vi "Updated4x7Display.vi"(8 "Error In":errorcluster, 10 "Cluster":cluster{"Score":u32, "Time":u32, "Combo":u32}={"Score"=4, "Time"=4, "Combo"=4}, 11 "LINX Resource In":T1) -> (0 "Error Out":errorcluster, 3 "LINX Resource Out":T1)   [LabVIEW 2022 SP3]
doc: "Custom Command 7 is for the Score Display. Custom Command 8 is for the Time Display. Custom Command 9 is for Combo Display. Sends number to display to the applicable 7 segment display."
uses:
  <vilib>/MakerHub/LINX/Private/Type Defs/LINX Ref.ctl
  <vilib>/MakerHub/LINX/Private/Type Defs/Platform.ctl
  <vilib>/MakerHub/LINX/Private/Type Defs/Interface.ctl
  <vilib>/MakerHub/LINX/Private/Device/Type Defs/LINX Device Config.ctl
  <vilib>/MakerHub/LINX/Private/Device/Type Defs/TCP Config.ctl
  <vilib>/MakerHub/LINX/Private/Device/Type Defs/Channels.ctl
  <vilib>/MakerHub/LINX/LMH-LINX.lvlib
  <vilib>/MakerHub/LINX/Private/Device/Device.lvlib
panel:
  out "Response":u8[](array[numeric])
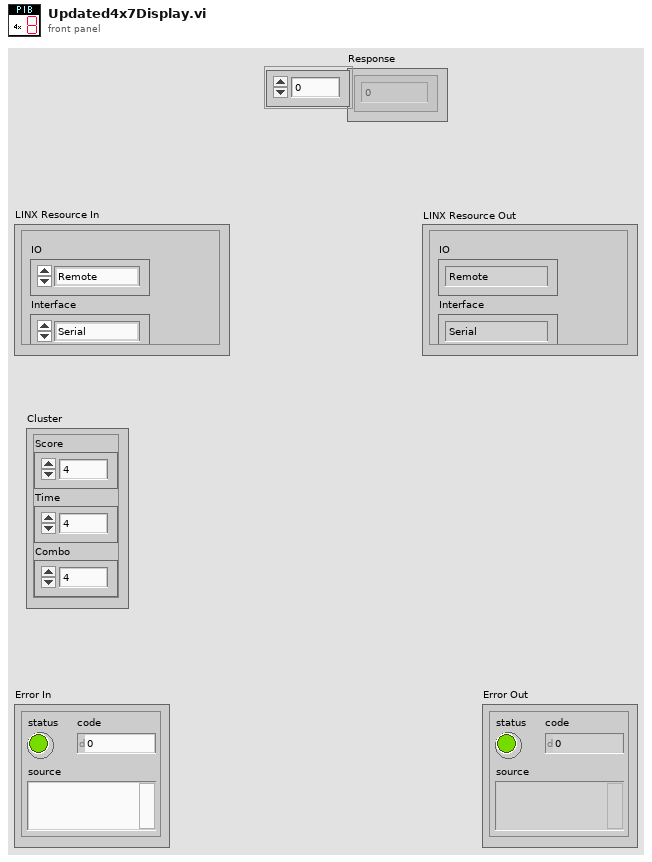
[diagram p1: front panel]
types:
  T1 = typedef "LMH-LINX.lvlib/LINX Ref.ctl" = cluster{"IO":T2, "Interface":T3, "LINX Device Config":T4}
  T2 = typedef "LMH-LINX.lvlib/Platform.ctl" = enum16{"Remote", "Local"}
  T3 = typedef "LMH-LINX.lvlib/Interface.ctl" = enum16{"Serial", "TCP"}
  T4 = typedef "LMH-LINX.lvlib/Device.lvlib/LINX Device Config.ctl" = cluster{"Interface":T3, "COM Port":refnum<visa-resource-name>, "TCP Configuration":T5, "Device Family":u8, "Device ID":u8, "Device Name":string, "TCP Ref":refnum<k5>, "Channels":T6}
  T5 = typedef "LMH-LINX.lvlib/Device.lvlib/TCP Config.ctl" = cluster{"IP Address":string, "Port":u16}
  T6 = typedef "LMH-LINX.lvlib/Channels.ctl" = cluster{"DI":u8[], "DO":u8[], "AI":u8[], "AO":u8[], "PWM":u8[], "QE":u8[], "UART":u8[], "I2C 2":u8[], "SPI":u8[], "CAN":u8[], "Servo":u8[], "AI Ref (V)":dbl, "AI Resolution (Bits)":u8, "AO Ref (V)":dbl, "AO Resolution (Bits)":u8}
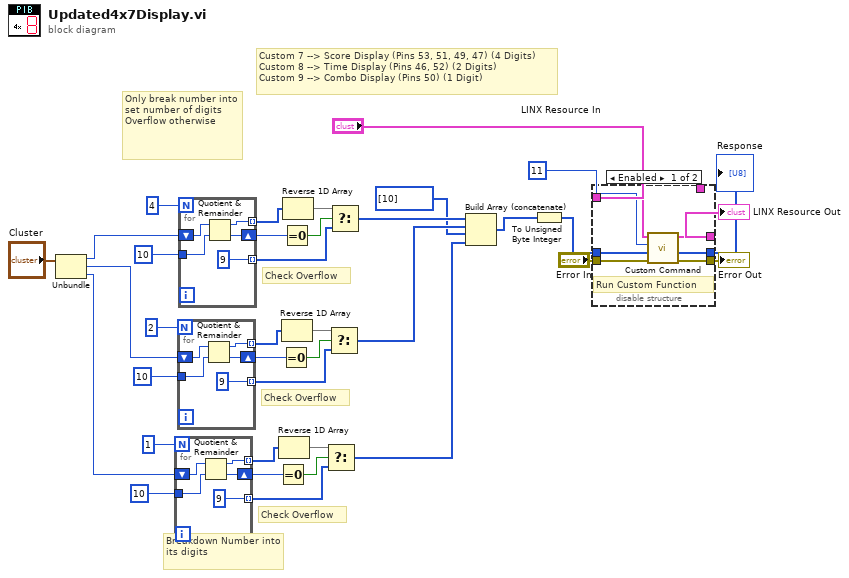
[diagram p0: block diagram]
diagram:
  # "Check Overflow"
  # "Check Overflow"
  # "Check Overflow"
  # "Breakdown Number into its digits"
  # "Custom 7 --> Score Display (Pins 53, 51, 49, 47) (4 Digits)\nCustom 8 --> Time Display (Pins 46, 52) (2 Digits)\nCustom 9 --> Combo Display (Pins 50) (1 Digit)"
  # "Only break number into set number of digits\nOverflow otherwise"
  n1 = Unbundle("Cluster") -> ("Score"=w31:u32, "Time"=w30:u32, "Combo"=w29:u32)
  n2 = for {
    N: 1 ("Display Length") -> [_]
    tunnel: u32 10 -> [w38]
    tunnel: [w40] -> w6 mode=indexing
    tunnel: [u32 9] -> w7 mode=indexing
    shift-right: [w41] -> w5
    shift-left: w29 -> [w42]
    n3 = Quotient & Remainder(x=w42, y=w38) -> (x-y*floor(x/y)=w40:u32, floor(x/y)=w41:u32)
  }
  n4 = for {
    N: 2 ("Display Length") -> [_]
    tunnel: u32 10 -> [w43]
    tunnel: [w45] -> w13 mode=indexing
    tunnel: [u32 9] -> w14 mode=indexing
    shift-right: [w46] -> w12
    shift-left: w30 -> [w47]
    n5 = Quotient & Remainder(x=w47, y=w43) -> (x-y*floor(x/y)=w45:u32, floor(x/y)=w46:u32)
  }
  n6 = for {
    N: 4 ("Display Length") -> [_]
    tunnel: u32 10 -> [w48]
    tunnel: [w50] -> w20 mode=indexing
    tunnel: [u32 9] -> w21 mode=indexing
    shift-right: [w51] -> w19
    shift-left: w31 -> [w52]
    n7 = Quotient & Remainder(x=w52, y=w48) -> (x-y*floor(x/y)=w50:u32, floor(x/y)=w51:u32)
  }
  n8 = Equal To 0?(x=w5) -> (x = 0?=w8:bool)
  n9 = Reverse 1D Array(array=w6) -> (reversed array=w9:u32[])
  n10 = Equal To 0?(x=w12) -> (x = 0?=w15:bool)
  n11 = Equal To 0?(x=w19) -> (x = 0?=w22:bool)
  n12 = Reverse 1D Array(array=w13) -> (reversed array=w16:u32[])
  n13 = Reverse 1D Array(array=w20) -> (reversed array=w23:u32[])
  n14 = Select(t=w9, s=w8, f=w7) -> (s? t:f=w2:u32[])
  n15 = Select(t=w16, s=w15, f=w14) -> (s? t:f=w24:u32[])
  n16 = Select(t=w23, s=w22, f=w21) -> (s? t:f=w25:u32[])
  n17 = Build Array (concatenate)(w25, w24, u32[] [10] ("array"), w2) -> (w28:u32[])
  n18 = To Unsigned Byte Integer(number=w28) -> (unsigned 8bit integer=w36:u8[])
  n19 = disable-structure shown="Enabled" {
    disable-tunnel: u16 11 ("Custom Command Number") -> [w59 _]
    disable-tunnel: w36 -> [w58 w61]
    disable-tunnel: "LINX Resource In" -> [w57 _]
    disable-tunnel: [w56 w62] -> w35
    disable-tunnel: "Error In" -> [w55 w60]
    disable-tunnel: [w54 w60] -> w33
    disable-tunnel: [w53 w61] -> w27
    disable-tunnel: "LINX Resource In" -> [_ w62]
    frame Enabled {
      # "Run Custom Function"
      n20 = call <vilib>:"Custom Command.vi"("Error In"=w55, "Data"=w58, "Custom Command Number"=w59, "LINX Resource"=w57) -> ("Error Out"=w54:errorcluster, "Response"=w53:u8[], "LINX Resource"=w56:T1)  [unwired: 4 in, 1 out]
    }
    frame Disabled {
    }
  }
  "LINX Resource Out" <- w35
  "Error Out" <- w33
  "Response" <- w27
